vi "Build Single JSON.vi"(8 "error in":errorcluster, 9 "Consumer?":bool, 10 "ChannelName":string, 11 "Single":variant) -> (0 "error out":errorcluster, 3 "Channel":T1)   [LabVIEW 2023, in "Utilities.lvlib"]
uses:
  Utilities.lvlib
  Channel.ctl
  <vilib>/Utility/Data Type/NI_Data Type.lvlib
panel:
  in  "Channel":T1
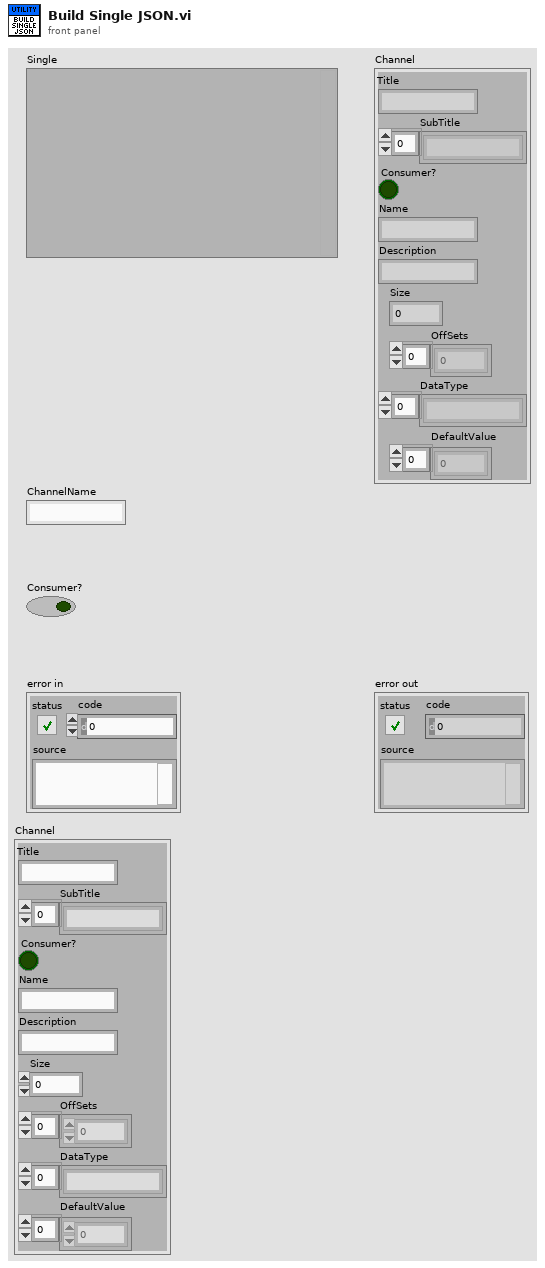
[diagram p1: front panel]
types:
  T1 = typedef "Utilities.lvlib/Channel.ctl" = cluster{"Title":string, "SubTitle":string[], "Consumer?":bool, "Name":string, "Description":string, "Size":i32, "OffSets":i32[], "DataType":string[], "DefaultValue":dbl[]}
  T2 = typedef "NI_Data Type.lvlib/Data Type.ctl" = enum8{"Invalid Type", "Void", "I8", "I16", "I32", "I64", "U8", "U16", "U32", "U64", "Single Float", "Double Float", "Extended Float", "Single Complex", "Double Complex", "Extended Complex", "Enum U8", "Enum U16", "Enum U32", "Enum U64", "Single Float With Unit", "Double Float With Unit", "Extended Float With Unit", "Single Complex with Unit", "Double Complex with Unit", "Extended Complex with Unit", "Boolean", "String", "Path", "Picture", "Tag", "Array", "Cluster", "Variant", "LV Variant", "Waveform", "Timestamp", "Digital Waveform", "Digital Data", "ExpressData", "Refnum", "External Data", "VI", "Poly VI", "LabVIEW Class Instance", "Fixed Point", "Set Collection", "Map Collection"}
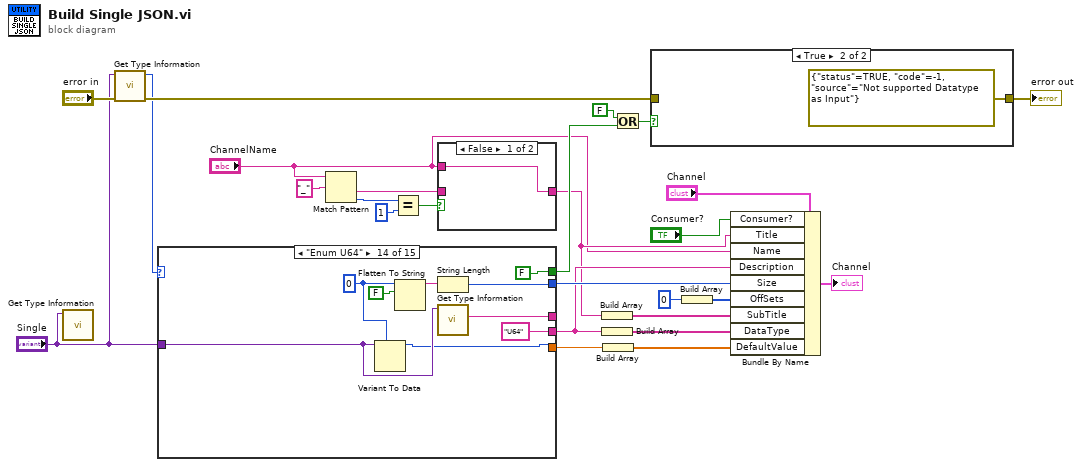
[diagram p0: block diagram]
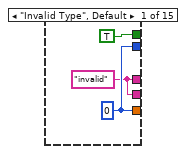
[diagram p3: hidden frame]
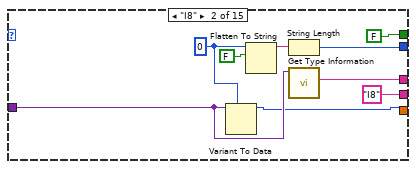
[diagram p4: hidden frame]
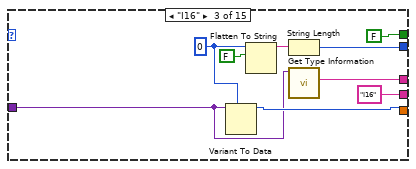
[diagram p5: hidden frame]
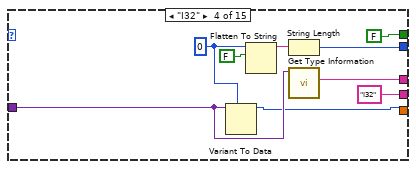
[diagram p6: hidden frame]
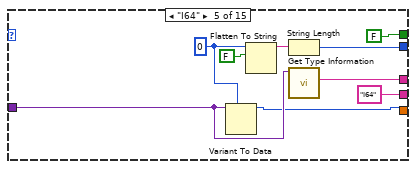
[diagram p7: hidden frame]
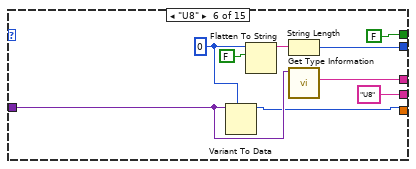
[diagram p8: hidden frame]
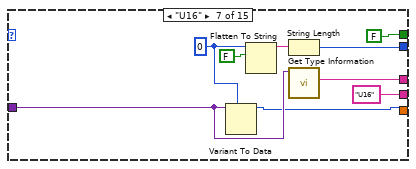
[diagram p9: hidden frame]
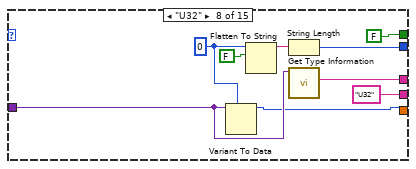
[diagram p10: hidden frame]
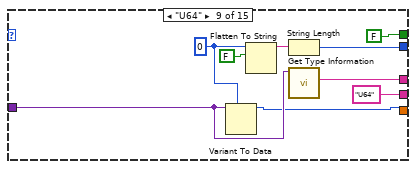
[diagram p11: hidden frame]
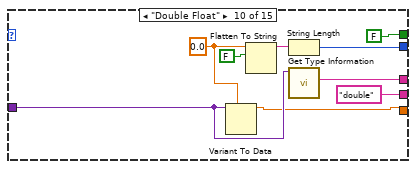
[diagram p12: hidden frame]
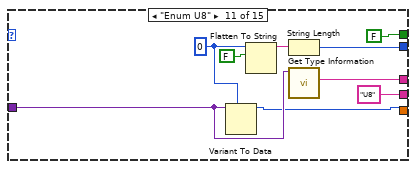
[diagram p13: hidden frame]
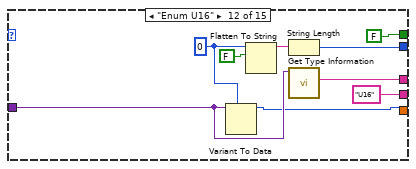
[diagram p14: hidden frame]
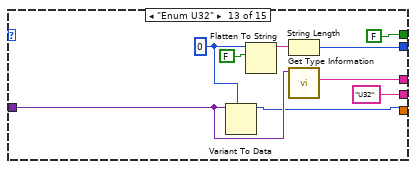
[diagram p15: hidden frame]
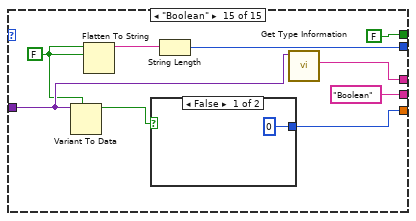
[diagram p16: hidden frame]
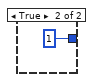
[diagram p17: hidden frame]
diagram:
  n1 = call <vilib>:"Get Type Information.vi"("variant"="Single") -> ()  [unwired: 6 in, 5 out]
  n2 = call <vilib>:"Get Type Information.vi"("error in (no error)"="error in", "variant"="Single") -> ("error out"=w23:errorcluster, "type"=w22:T2)  [unwired: 5 in, 3 out]
  n3 = case shown="\"Enum U64\"" w22 {
    tunnel: [TRUE FALSE FALSE FALSE FALSE FALSE FALSE FALSE FALSE FALSE FALSE FALSE FALSE FALSE FALSE] -> w21
    tunnel: [w28 w36 w45 w54 w63 w72 w81 w90 w99 w108 w117 w126 w135 w143 w153] -> w11
    tunnel: "Single" -> [_ w32 w40 w50 w59 w68 w77 w86 w95 w104 w113 w122 w131 w140 w150]
    tunnel: [w27 w34 w42 w51 w60 w70 w78 w87 w96 w106 w114 w123 w132 w141 w151] -> _
    tunnel: [w27 "I8" "I16" "I32" "I64" "U8" "U16" "U32" "U64" "double" "U8" "U16" "U32" "U64" "Boolean"] -> w10
    tunnel: [w28 w30 w41 w48 w57 w66 w75 w85 w93 w102 w111 w120 w130 w138 w147] -> w2
    frame "Invalid Type", Default {
      w27 = "invalid" ("name")
      w28 = 0
    }
    frame "I8" {
      w31 = i8 0
      n4 = Variant To Data(type=w31, Variant=w32) -> (data=w30:i8)  [unwired: 1 in, 1 out]
      n5 = Flatten To String(anything=w31, prepend array or string size? (T)=FALSE) -> (data string=w37:string)  [unwired: 2 in, 2 out]
      n6 = String Length(string=w37) -> (length=w36:i32)
      n7 = call <vilib>:"Get Type Information.vi"("variant"=w32) -> ("name"=w34:string)  [unwired: 6 in, 4 out]
    }
    frame "I16" {
      w39 = i16 0
      n8 = Variant To Data(type=w39, Variant=w40) -> (data=w41:i16)  [unwired: 1 in, 1 out]
      n9 = Flatten To String(anything=w39, prepend array or string size? (T)=FALSE) -> (data string=w46:string)  [unwired: 2 in, 2 out]
      n10 = String Length(string=w46) -> (length=w45:i32)
      n11 = call <vilib>:"Get Type Information.vi"("variant"=w40) -> ("name"=w42:string)  [unwired: 6 in, 4 out]
    }
    frame "I32" {
      w49 = 0
      n12 = Variant To Data(type=w49, Variant=w50) -> (data=w48:i32)  [unwired: 1 in, 1 out]
      n13 = Flatten To String(anything=w49, prepend array or string size? (T)=FALSE) -> (data string=w55:string)  [unwired: 2 in, 2 out]
      n14 = String Length(string=w55) -> (length=w54:i32)
      n15 = call <vilib>:"Get Type Information.vi"("variant"=w50) -> ("name"=w51:string)  [unwired: 6 in, 4 out]
    }
    frame "I64" {
      w58 = i64 0
      n16 = Variant To Data(type=w58, Variant=w59) -> (data=w57:i64)  [unwired: 1 in, 1 out]
      n17 = Flatten To String(anything=w58, prepend array or string size? (T)=FALSE) -> (data string=w64:string)  [unwired: 2 in, 2 out]
      n18 = String Length(string=w64) -> (length=w63:i32)
      n19 = call <vilib>:"Get Type Information.vi"("variant"=w59) -> ("name"=w60:string)  [unwired: 6 in, 4 out]
    }
    frame "U8" {
      w67 = u8 0
      n20 = Variant To Data(type=w67, Variant=w68) -> (data=w66:u8)  [unwired: 1 in, 1 out]
      n21 = Flatten To String(anything=w67, prepend array or string size? (T)=FALSE) -> (data string=w73:string)  [unwired: 2 in, 2 out]
      n22 = String Length(string=w73) -> (length=w72:i32)
      n23 = call <vilib>:"Get Type Information.vi"("variant"=w68) -> ("name"=w70:string)  [unwired: 6 in, 4 out]
    }
    frame "U16" {
      w76 = u16 0
      n24 = Variant To Data(type=w76, Variant=w77) -> (data=w75:u16)  [unwired: 1 in, 1 out]
      n25 = Flatten To String(anything=w76, prepend array or string size? (T)=FALSE) -> (data string=w82:string)  [unwired: 2 in, 2 out]
      n26 = String Length(string=w82) -> (length=w81:i32)
      n27 = call <vilib>:"Get Type Information.vi"("variant"=w77) -> ("name"=w78:string)  [unwired: 6 in, 4 out]
    }
    frame "U32" {
      w84 = u32 0
      n28 = Variant To Data(type=w84, Variant=w86) -> (data=w85:u32)  [unwired: 1 in, 1 out]
      n29 = Flatten To String(anything=w84, prepend array or string size? (T)=FALSE) -> (data string=w91:string)  [unwired: 2 in, 2 out]
      n30 = String Length(string=w91) -> (length=w90:i32)
      n31 = call <vilib>:"Get Type Information.vi"("variant"=w86) -> ("name"=w87:string)  [unwired: 6 in, 4 out]
    }
    frame "U64" {
      w94 = u64 0
      n32 = Variant To Data(type=w94, Variant=w95) -> (data=w93:u64)  [unwired: 1 in, 1 out]
      n33 = Flatten To String(anything=w94, prepend array or string size? (T)=FALSE) -> (data string=w100:string)  [unwired: 2 in, 2 out]
      n34 = String Length(string=w100) -> (length=w99:i32)
      n35 = call <vilib>:"Get Type Information.vi"("variant"=w95) -> ("name"=w96:string)  [unwired: 6 in, 4 out]
    }
    frame "Double Float" {
      w103 = 0.0
      n36 = Variant To Data(type=w103, Variant=w104) -> (data=w102:dbl)  [unwired: 1 in, 1 out]
      n37 = Flatten To String(anything=w103, prepend array or string size? (T)=FALSE) -> (data string=w109:string)  [unwired: 2 in, 2 out]
      n38 = String Length(string=w109) -> (length=w108:i32)
      n39 = call <vilib>:"Get Type Information.vi"("variant"=w104) -> ("name"=w106:string)  [unwired: 6 in, 4 out]
    }
    frame "Enum U8" {
      w112 = u8 0
      n40 = Variant To Data(type=w112, Variant=w113) -> (data=w111:u8)  [unwired: 1 in, 1 out]
      n41 = Flatten To String(anything=w112, prepend array or string size? (T)=FALSE) -> (data string=w118:string)  [unwired: 2 in, 2 out]
      n42 = String Length(string=w118) -> (length=w117:i32)
      n43 = call <vilib>:"Get Type Information.vi"("variant"=w113) -> ("name"=w114:string)  [unwired: 6 in, 4 out]
    }
    frame "Enum U16" {
      w121 = u16 0
      n44 = Variant To Data(type=w121, Variant=w122) -> (data=w120:u16)  [unwired: 1 in, 1 out]
      n45 = Flatten To String(anything=w121, prepend array or string size? (T)=FALSE) -> (data string=w127:string)  [unwired: 2 in, 2 out]
      n46 = String Length(string=w127) -> (length=w126:i32)
      n47 = call <vilib>:"Get Type Information.vi"("variant"=w122) -> ("name"=w123:string)  [unwired: 6 in, 4 out]
    }
    frame "Enum U32" {
      w129 = u32 0
      n48 = Variant To Data(type=w129, Variant=w131) -> (data=w130:u32)  [unwired: 1 in, 1 out]
      n49 = Flatten To String(anything=w129, prepend array or string size? (T)=FALSE) -> (data string=w136:string)  [unwired: 2 in, 2 out]
      n50 = String Length(string=w136) -> (length=w135:i32)
      n51 = call <vilib>:"Get Type Information.vi"("variant"=w131) -> ("name"=w132:string)  [unwired: 6 in, 4 out]
    }
    frame "Enum U64" {
      w139 = u64 0
      n52 = Variant To Data(type=w139, Variant=w140) -> (data=w138:u64)  [unwired: 1 in, 1 out]
      n53 = Flatten To String(anything=w139, prepend array or string size? (T)=FALSE) -> (data string=w145:string)  [unwired: 2 in, 2 out]
      n54 = String Length(string=w145) -> (length=w143:i32)
      n55 = call <vilib>:"Get Type Information.vi"("variant"=w140) -> ("name"=w141:string)  [unwired: 6 in, 4 out]
    }
    frame "Boolean" {
      w149 = FALSE ("prepend array or string size? (T)")
      n56 = Variant To Data(type=w149, Variant=w150) -> (data=w148:bool)  [unwired: 1 in, 1 out]
      n57 = Flatten To String(anything=w149, prepend array or string size? (T)=w149) -> (data string=w155:string)  [unwired: 2 in, 2 out]
      n58 = case shown="False" w148 {
        tunnel: [0 1] -> w147
        frame False {
        }
        frame True {
        }
      }
      n59 = String Length(string=w155) -> (length=w153:i32)
      n60 = call <vilib>:"Get Type Information.vi"("variant"=w150) -> ("name"=w151:string)  [unwired: 6 in, 4 out]
    }
  }
  n61 = Match Pattern(string="ChannelName", regular expression="_") -> (after substring=w8:string, offset past match=w7:i32)  [unwired: 1 in, 2 out]
  n62 = Equal?(x=w7, y=1) -> (x = y?=w5:bool)
  n63 = case shown="False" w5 {
    tunnel: "ChannelName" -> [w158 _]
    tunnel: [w158 w159] -> w4
    tunnel: w8 -> [_ w159]
    frame False {
    }
    frame True {
    }
  }
  n64 = Build Array(w4) -> (w14:string[])
  n65 = Build Array(w10) -> (w13:string[])
  n66 = Build Array(w2) -> (w1:dbl[])
  n67 = Or(x=FALSE, y=w21) -> (x .or. y?=w25:bool)
  n68 = case shown="True" w25 {
    tunnel: w23 -> [w160 _]
    tunnel: [w160 errorcluster {"status"=TRUE, "code"=-1, "source"="Not supported Datatype as Input"} ("error in")] -> w24
    frame False {
    }
    frame True {
    }
  }
  "error out" <- w24
  n69 = Build Array(0 ("element")) -> (w12:i32[])
  n70 = Bundle By Name(cluster="Channel", "Consumer?"="Consumer?", "Title"=w4, "Name"="ChannelName", "Description"=w10, "Size"=w11, "OffSets"=w12, "SubTitle"=w14, "DataType"=w13, "DefaultValue"=w1) -> (→"Channel":T1)
